vi "Read X.vi"(8 "error in (no error)":errorcluster, 11 "VISA Refnum in":refnum<visa-resource-name>) -> (0 "error out":errorcluster, 1 "Return Data Bytes":u16, 2 "Return All Data":string, 3 "VISA Refnum out":refnum<visa-resource-name>, 5 "Wavelike Data":dbl[](array[numeric]))   [LabVIEW 2021]
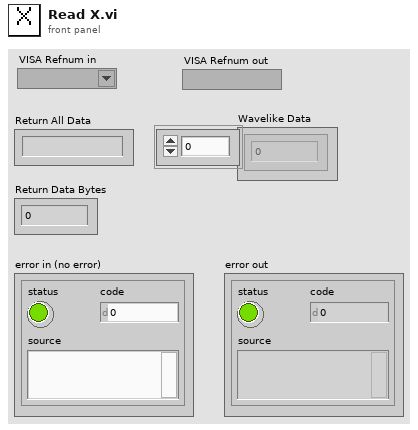
[diagram p1: front panel]
types:
  T1 = enum16{"Y AXIS Data Output", "X AXIS Data Output"}
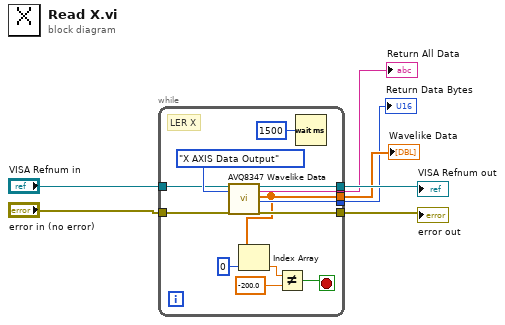
[diagram p0: block diagram]
diagram:
  n1 = while {
    tunnel: [w19] -> w1
    tunnel: [w18] -> w2
    tunnel: [w10] -> w3
    tunnel: "VISA Refnum in" -> [w15]
    tunnel: [w17] -> w6
    tunnel: "error in (no error)" -> [w14]
    tunnel: [w16] -> w7
    stop <- w8 stop-if-true
    # "LER X"
    n2 = call "AVQ8347 Wavelike Data.vi"("VISA Session"=w15, "Axis Select"=T1."X AXIS Data Output", "Error In"=w14) -> ("Copy VISA Session"=w17:refnum<visa-resource-name>, "Return All Data"=w19:string, "Wavelike Data"=w10:dbl[], "Return Data Bytes"=w18:u16, "Error Out"=w16:errorcluster)  [unwired: 12 in]
    n3 = Index Array(array=w10, index=0) -> (element=w9:dbl)
    n4 = Not Equal?(x=w9, y=-200.0) -> (x != y?=w8:bool)
    n5 = Wait (ms)(milliseconds to wait=u32 1500) -> ()  [unwired: 1 out]
  }
  "error out" <- w7
  "VISA Refnum out" <- w6
  "Wavelike Data" <- w3
  "Return Data Bytes" <- w2
  "Return All Data" <- w1
